vi "Read Created Timestamp.vi"(8 "error in (no error)":errorcluster, 11 "Oauth2.GitLab in":refnum<class "Oauth2.GitLab.lvclass">) -> (0 "error out":errorcluster, 2 "Created At":timestamp, 3 "Oauth2.GitLab out":refnum<class "Oauth2.GitLab.lvclass">)   [LabVIEW 2013, in "Oauth2.GitLab.lvclass"]
uses:
  Oauth2.GitLab.lvclass
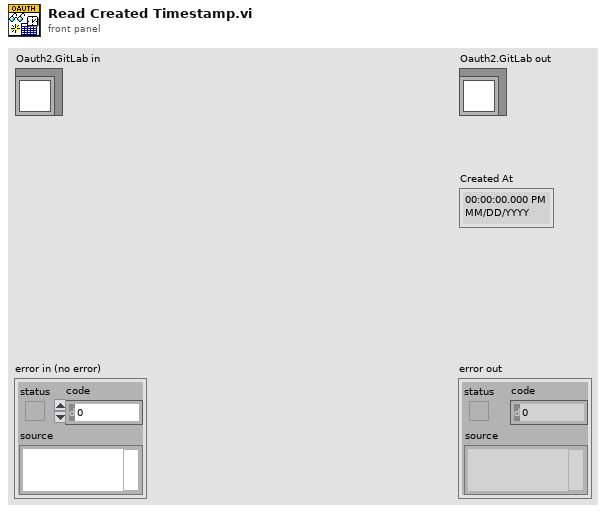
[diagram p1: front panel]
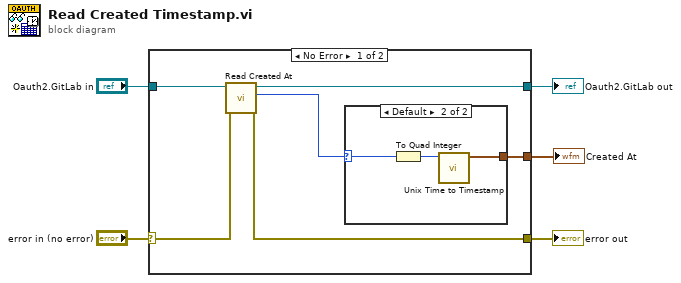
[diagram p0: block diagram]
diagram:
  n1 = case shown="No Error" "error in (no error)" {
    selector: "error in (no error)" -> [w10 w16]
    tunnel: [w9 w16] -> w4
    tunnel: [w8 w15] -> w2
    tunnel: "Oauth2.GitLab in" -> [w11 w15]
    tunnel: [w7 _] -> w1
    frame No Error {
      n2 = call "Read Created At.vi"("error in (no error)"=w10, "Oauth2.GitLab in"=w11) -> ("error out"=w9:errorcluster, "Created At"=w6:u32, "Oauth2.GitLab out"=w8:refnum<class "Oauth2.GitLab.lvclass">)  [unwired: 7 in]
      n3 = case shown="Default" w6 {
        selector: w6 -> [_ w12]
        tunnel: [_ w13] -> w7
        frame 0 {
        }
        frame Default {
          n4 = To Quad Integer(1:w12) -> (0:w14:i64)
          n5 = call <vilib>:"Unix Time to Timestamp.vi"("Unix Time (s)"=w14) -> ("Timestamp"=w13:timestamp)  [unwired: 9 in, 1 out]
        }
      }
    }
    frame Error {
    }
  }
  "error out" <- w4
  "Oauth2.GitLab out" <- w2
  "Created At" <- w1
